vi "ItWorks.vi"(5 "strMessage":string) -> ()   [LabVIEW 2011]
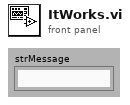
[diagram p1: front panel]
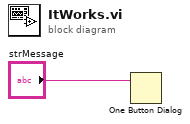
[diagram p0: block diagram]
diagram:
  n1 = One Button Dialog(message="strMessage") -> ()  [unwired: 2 out]
